vi "Extract subclasses from temperature device.vi"(9 "Data In":string, 10 "Class":string, 11 "Temperature Device Settings in":T1) -> (1 "Data out":string, 3 "Temperature Device Settings out":T1)   [LabVIEW 2014, in "Mercury iXX.lvlib" / "Temperature.lvlib"]
uses:
  Temperature.lvlib
  Controls/Temperature Device (Read).ctl
  Controls/Manufacturing Data.ctl
  Controls/Temperature Sensor Type.ctl
  Controls/Excitation Cluster.ctl
  Controls/Excitation Type.ctl
  Controls/Calibration Cluster.ctl
  Controls/Calibration Interpolation.ctl
  Controls/Loop Cluster.ctl
  Controls/Temperature Signals Cluster.ctl
  Mercury iXX.lvlib
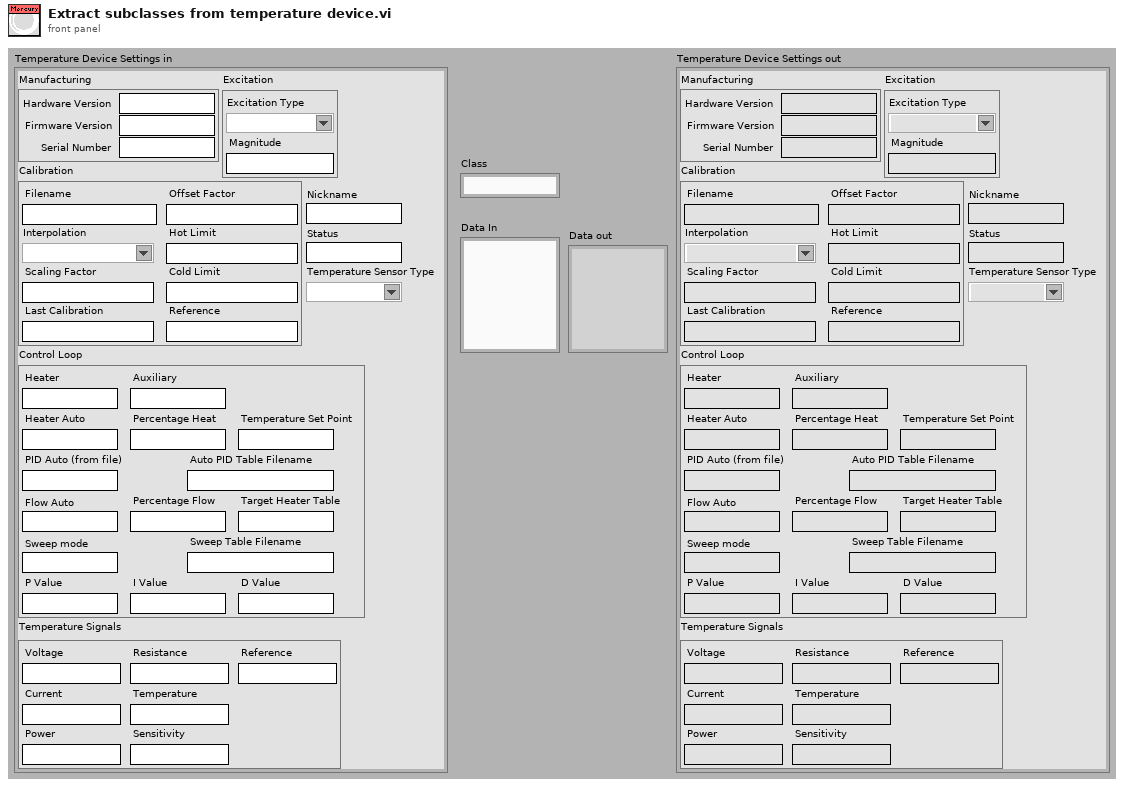
[diagram p1: front panel]
types:
  T1 = typedef "Mercury iXX.lvlib/Temperature.lvlib/Temperature Device (Read).ctl" = cluster{"Manufacturing":T2, "Temperature Sensor Type":T3, "Excitation":T4, "Calibration":T6, "Control Loop":T8, "Temperature Signals":T9, "Nickname":string, "Status":string}
  T2 = typedef "Mercury iXX.lvlib/Manufacturing Data.ctl" = cluster{"Hardware Version":string, "Firmware Version":string, "Serial Number":string}
  T3 = typedef "Mercury iXX.lvlib/Temperature.lvlib/Temperature Sensor Type.ctl" = string
  T4 = typedef "Mercury iXX.lvlib/Temperature.lvlib/Excitation Cluster.ctl" = cluster{"Excitation Type":T5, "Magnitude":string}
  T5 = typedef "Mercury iXX.lvlib/Temperature.lvlib/Excitation Type.ctl" = string
  T6 = typedef "Mercury iXX.lvlib/Temperature.lvlib/Calibration Cluster.ctl" = cluster{"Filename":string, "Interpolation":T7, "Scaling Factor":string, "Offset Factor":string, "Hot Limit":string, "Cold Limit":string, "Last Calibration":string, "Reference":string}
  T7 = typedef "Mercury iXX.lvlib/Temperature.lvlib/Calibration Interpolation.ctl" = string
  T8 = typedef "Mercury iXX.lvlib/Temperature.lvlib/Loop Cluster.ctl" = cluster{"Heater":string, "Auxiliary":string, "Heater Auto":string, "Percentage Heat":string, "Temperature Set Point":string, "PID Auto (from file)":string, "P Value":string, "I Value":string, "D Value":string, "Auto PID Table Filename":string, "Flow Auto":string, "Target Heater Table":string, "Sweep mode":string, "Sweep Table Filename":string, "Percentage Flow":string}
  T9 = typedef "Mercury iXX.lvlib/Temperature.lvlib/Temperature Signals Cluster.ctl" = cluster{"Voltage":string, "Current":string, "Power":string, "Resistance":string, "Temperature":string, "Sensitivity":string, "Reference":string}
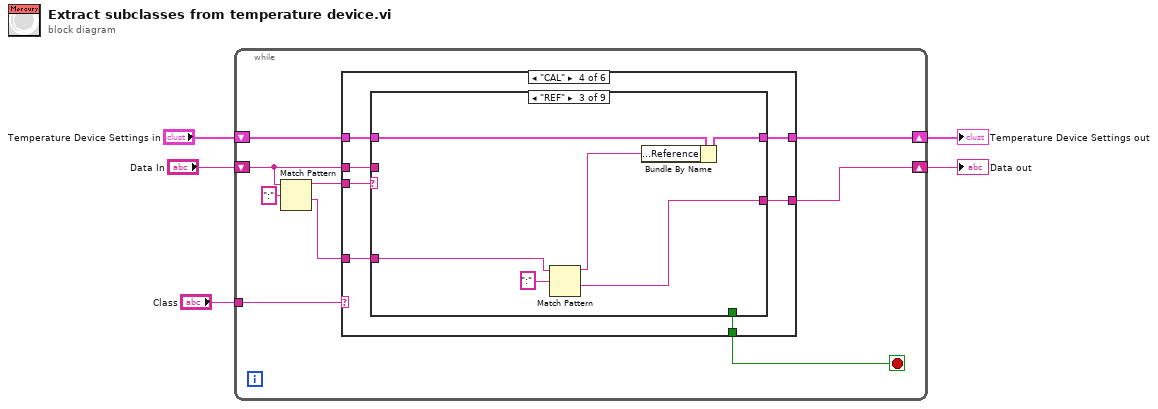
[diagram p0: block diagram]
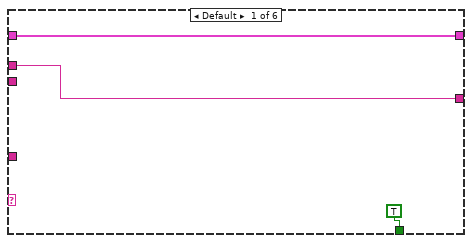
[diagram p2: hidden frame]
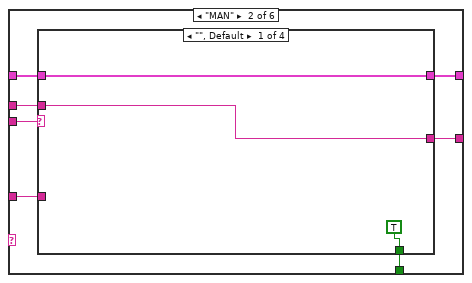
[diagram p3: hidden frame]
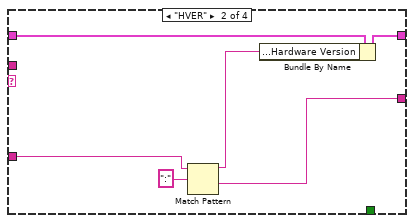
[diagram p4: hidden frame]
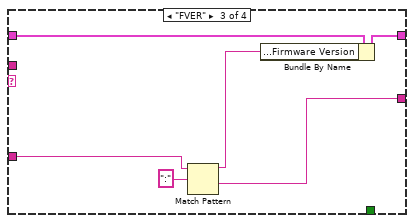
[diagram p5: hidden frame]
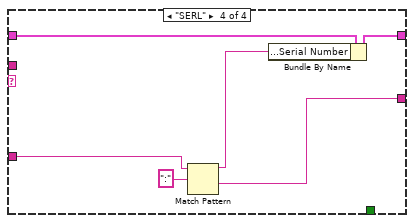
[diagram p6: hidden frame]
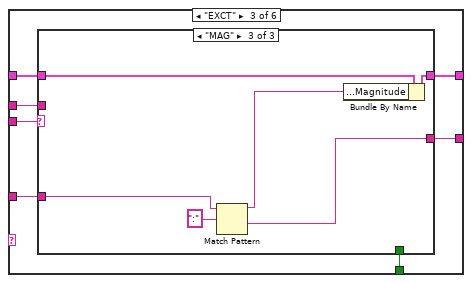
[diagram p7: hidden frame]
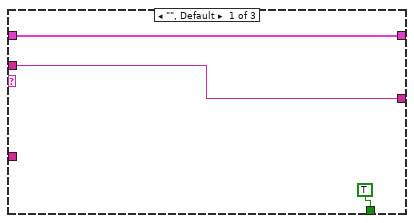
[diagram p8: hidden frame]
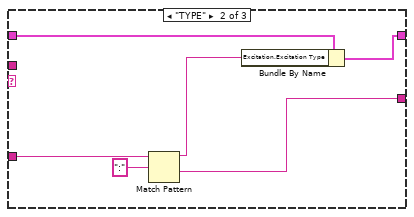
[diagram p9: hidden frame]
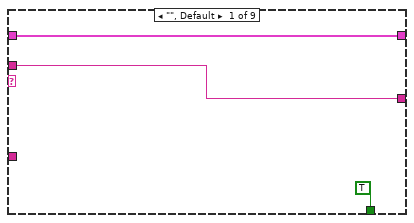
[diagram p10: hidden frame]
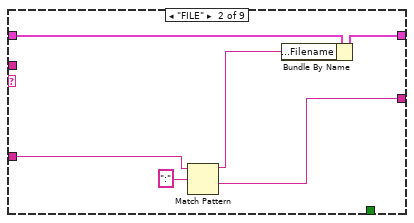
[diagram p11: hidden frame]
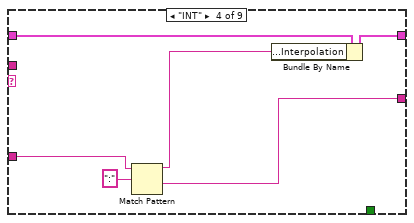
[diagram p12: hidden frame]
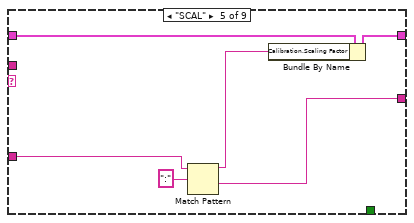
[diagram p13: hidden frame]
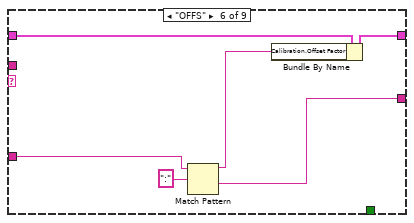
[diagram p14: hidden frame]
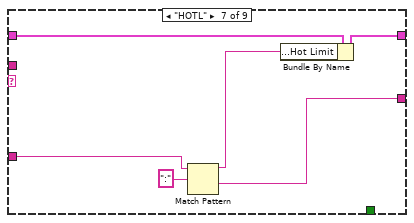
[diagram p15: hidden frame]
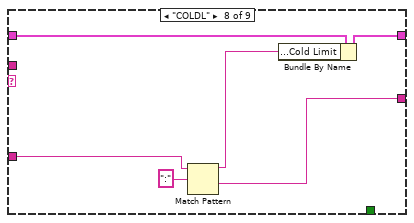
[diagram p16: hidden frame]
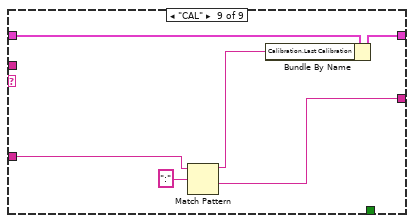
[diagram p17: hidden frame]
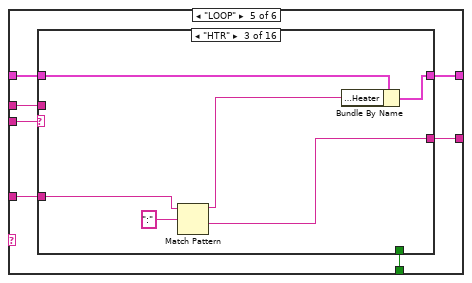
[diagram p18: hidden frame]
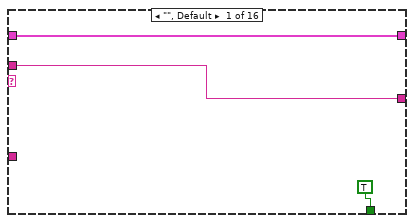
[diagram p19: hidden frame]
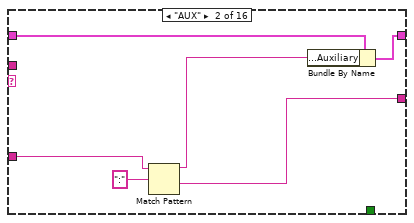
[diagram p20: hidden frame]
diagram:
  n1 = while {
    tunnel: "Class" -> [w7]
    shift-right: [w10] -> w4
    shift-left: "Data In" -> [w8]
    shift-right: [w12] -> w3
    shift-left: "Temperature Device Settings in" -> [w13]
    stop <- w6 stop-if-true
    n2 = Match Pattern(string=w8, regular expression=":") -> (before substring=w9:string, after substring=w11:string)  [unwired: 3 out]
    n3 = case shown="\"CAL\"" w7 {
      tunnel: w13 -> [w17 w24 w52 w74 w132 w232]
      tunnel: [w17 w23 w51 w73 w131 w231] -> w12
      tunnel: w11 -> [_ w22 w50 w72 w130 w230]
      tunnel: [w16 w21 w49 w71 w129 w229] -> w10
      tunnel: w9 -> [_ w20 w48 w70 w128 w228]
      tunnel: w8 -> [w16 w19 w47 w69 w127 w227]
      tunnel: [TRUE w18 w46 w68 w126 w226] -> w6
      frame Default {
      }
      frame "MAN" {
        n4 = case shown="\"\", Default" w20 {
          tunnel: w24 -> [w27 w33 w39 w45]
          tunnel: [w27 w32 w38 w44] -> w23
          tunnel: w22 -> [_ w31 w37 w43]
          tunnel: [w26 w30 w36 w42] -> w21
          tunnel: w19 -> [w26 _ _ _]
          tunnel: [TRUE _ _ _] -> w18
          frame "", Default {
          }
          frame "HVER" {
            n5 = Match Pattern(string=w31, regular expression=":") -> (before substring=w28:string, after substring=w30:string)  [unwired: 3 out]
            n6 = Bundle By Name(cluster=w33, "Manufacturing.Hardware Version"=w28) -> (w32:T1)
          }
          frame "FVER" {
            n7 = Match Pattern(string=w37, regular expression=":") -> (before substring=w34:string, after substring=w36:string)  [unwired: 3 out]
            n8 = Bundle By Name(cluster=w39, "Manufacturing.Firmware Version"=w34) -> (w38:T1)
          }
          frame "SERL" {
            n9 = Match Pattern(string=w43, regular expression=":") -> (before substring=w40:string, after substring=w42:string)  [unwired: 3 out]
            n10 = Bundle By Name(cluster=w45, "Manufacturing.Serial Number"=w40) -> (w44:T1)
          }
        }
      }
      frame "EXCT" {
        n11 = case shown="\"MAG\"" w48 {
          tunnel: w52 -> [w55 w61 w67]
          tunnel: [w55 w60 w66] -> w51
          tunnel: w50 -> [_ w58 w65]
          tunnel: [w54 w57 w64] -> w49
          tunnel: w47 -> [w54 _ _]
          tunnel: [TRUE _ _] -> w46
          frame "", Default {
          }
          frame "TYPE" {
            n12 = Match Pattern(string=w58, regular expression=":") -> (before substring=w56:string, after substring=w57:string)  [unwired: 3 out]
            n13 = Bundle By Name(cluster=w61, "Excitation.Excitation Type"=w56) -> (w60:T1)
          }
          frame "MAG" {
            n14 = Match Pattern(string=w65, regular expression=":") -> (before substring=w62:string, after substring=w64:string)  [unwired: 3 out]
            n15 = Bundle By Name(cluster=w67, "Excitation.Magnitude"=w62) -> (w66:T1)
          }
        }
      }
      frame "CAL" {
        n16 = case shown="\"REF\"" w70 {
          tunnel: w74 -> [w77 w83 w89 w95 w101 w107 w113 w119 w125]
          tunnel: [w77 w82 w88 w94 w100 w106 w112 w118 w124] -> w73
          tunnel: w72 -> [_ w81 w87 w93 w99 w105 w111 w117 w123]
          tunnel: [w76 w80 w86 w92 w98 w104 w110 w116 w122] -> w71
          tunnel: w69 -> [w76 _ _ _ _ _ _ _ _]
          tunnel: [TRUE _ _ _ _ _ _ _ _] -> w68
          frame "", Default {
          }
          frame "FILE" {
            n17 = Match Pattern(string=w81, regular expression=":") -> (before substring=w78:string, after substring=w80:string)  [unwired: 3 out]
            n18 = Bundle By Name(cluster=w83, "Calibration.Filename"=w78) -> (w82:T1)
          }
          frame "REF" {
            n19 = Match Pattern(string=w87, regular expression=":") -> (before substring=w84:string, after substring=w86:string)  [unwired: 3 out]
            n20 = Bundle By Name(cluster=w89, "Calibration.Reference"=w84) -> (w88:T1)
          }
          frame "INT" {
            n21 = Match Pattern(string=w93, regular expression=":") -> (before substring=w90:string, after substring=w92:string)  [unwired: 3 out]
            n22 = Bundle By Name(cluster=w95, "Calibration.Interpolation"=w90) -> (w94:T1)
          }
          frame "SCAL" {
            n23 = Match Pattern(string=w99, regular expression=":") -> (before substring=w96:string, after substring=w98:string)  [unwired: 3 out]
            n24 = Bundle By Name(cluster=w101, "Calibration.Scaling Factor"=w96) -> (w100:T1)
          }
          frame "OFFS" {
            n25 = Match Pattern(string=w105, regular expression=":") -> (before substring=w102:string, after substring=w104:string)  [unwired: 3 out]
            n26 = Bundle By Name(cluster=w107, "Calibration.Offset Factor"=w102) -> (w106:T1)
          }
          frame "HOTL" {
            n27 = Match Pattern(string=w111, regular expression=":") -> (before substring=w108:string, after substring=w110:string)  [unwired: 3 out]
            n28 = Bundle By Name(cluster=w113, "Calibration.Hot Limit"=w108) -> (w112:T1)
          }
          frame "COLDL" {
            n29 = Match Pattern(string=w117, regular expression=":") -> (before substring=w114:string, after substring=w116:string)  [unwired: 3 out]
            n30 = Bundle By Name(cluster=w119, "Calibration.Cold Limit"=w114) -> (w118:T1)
          }
          frame "CAL" {
            n31 = Match Pattern(string=w123, regular expression=":") -> (before substring=w120:string, after substring=w122:string)  [unwired: 3 out]
            n32 = Bundle By Name(cluster=w125, "Calibration.Last Calibration"=w120) -> (w124:T1)
          }
        }
      }
      frame "LOOP" {
        n33 = case shown="\"HTR\"" w128 {
          tunnel: w132 -> [w135 w141 w147 w153 w159 w165 w171 w177 w183 w189 w195 w201 w207 w213 w219 w225]
          tunnel: [w135 w140 w146 w152 w158 w164 w170 w176 w182 w188 w194 w200 w206 w212 w218 w224] -> w131
          tunnel: w130 -> [_ w138 w144 w150 w156 w162 w168 w174 w181 w187 w193 w199 w205 w211 w217 w223]
          tunnel: [w134 w137 w143 w149 w155 w161 w167 w173 w180 w186 w192 w198 w204 w210 w216 w222] -> w129
          tunnel: w127 -> [w134 _ _ _ _ _ _ _ _ _ _ _ _ _ _ _]
          tunnel: [TRUE _ _ _ _ _ _ _ _ _ _ _ _ _ _ _] -> w126
          frame "", Default {
          }
          frame "AUX" {
            n34 = Match Pattern(string=w138, regular expression=":") -> (before substring=w136:string, after substring=w137:string)  [unwired: 3 out]
            n35 = Bundle By Name(cluster=w141, "Control Loop.Auxiliary"=w136) -> (w140:T1)
          }
          frame "HTR" {
            n36 = Match Pattern(string=w144, regular expression=":") -> (before substring=w142:string, after substring=w143:string)  [unwired: 3 out]
            n37 = Bundle By Name(cluster=w147, "Control Loop.Heater"=w142) -> (w146:T1)
          }
          frame "ENAB" {
            n38 = Match Pattern(string=w150, regular expression=":") -> (before substring=w148:string, after substring=w149:string)  [unwired: 3 out]
            n39 = Bundle By Name(cluster=w153, "Control Loop.Heater Auto"=w148) -> (w152:T1)
          }
          frame "HSET" {
            n40 = Match Pattern(string=w156, regular expression=":") -> (before substring=w154:string, after substring=w155:string)  [unwired: 3 out]
            n41 = Bundle By Name(cluster=w159, "Control Loop.Percentage Heat"=w154) -> (w158:T1)
          }
          frame "TSET" {
            n42 = Match Pattern(string=w162, regular expression=":") -> (before substring=w160:string, after substring=w161:string)  [unwired: 3 out]
            n43 = Bundle By Name(cluster=w165, "Control Loop.Temperature Set Point"=w160) -> (w164:T1)
          }
          frame "PIDT" {
            n44 = Match Pattern(string=w168, regular expression=":") -> (before substring=w166:string, after substring=w167:string)  [unwired: 3 out]
            n45 = Bundle By Name(cluster=w171, "Control Loop.PID Auto (from file)"=w166) -> (w170:T1)
          }
          frame "PIDF" {
            n46 = Match Pattern(string=w174, regular expression=":") -> (before substring=w172:string, after substring=w173:string)  [unwired: 3 out]
            n47 = Bundle By Name(cluster=w177, "Control Loop.Auto PID Table Filename"=w172) -> (w176:T1)
          }
          frame "P" {
            n48 = Match Pattern(string=w181, regular expression=":") -> (before substring=w178:string, after substring=w180:string)  [unwired: 3 out]
            n49 = Bundle By Name(cluster=w183, "Control Loop.P Value"=w178) -> (w182:T1)
          }
          frame "I" {
            n50 = Match Pattern(string=w187, regular expression=":") -> (before substring=w184:string, after substring=w186:string)  [unwired: 3 out]
            n51 = Bundle By Name(cluster=w189, "Control Loop.I Value"=w184) -> (w188:T1)
          }
          frame "D" {
            n52 = Match Pattern(string=w193, regular expression=":") -> (before substring=w190:string, after substring=w192:string)  [unwired: 3 out]
            n53 = Bundle By Name(cluster=w195, "Control Loop.D Value"=w190) -> (w194:T1)
          }
          frame "FAUT" {
            n54 = Match Pattern(string=w199, regular expression=":") -> (before substring=w196:string, after substring=w198:string)  [unwired: 3 out]
            n55 = Bundle By Name(cluster=w201, "Control Loop.Flow Auto"=w196) -> (w200:T1)
          }
          frame "FSET" {
            n56 = Match Pattern(string=w205, regular expression=":") -> (before substring=w202:string, after substring=w204:string)  [unwired: 3 out]
            n57 = Bundle By Name(cluster=w207, "Control Loop.Percentage Flow"=w202) -> (w206:T1)
          }
          frame "THTF" {
            n58 = Match Pattern(string=w211, regular expression=":") -> (before substring=w208:string, after substring=w210:string)  [unwired: 3 out]
            n59 = Bundle By Name(cluster=w213, "Control Loop.Target Heater Table"=w208) -> (w212:T1)
          }
          frame "SWMD" {
            n60 = Match Pattern(string=w217, regular expression=":") -> (before substring=w214:string, after substring=w216:string)  [unwired: 3 out]
            n61 = Bundle By Name(cluster=w219, "Control Loop.Sweep mode"=w214) -> (w218:T1)
          }
          frame "SWFL" {
            n62 = Match Pattern(string=w223, regular expression=":") -> (before substring=w220:string, after substring=w222:string)  [unwired: 3 out]
            n63 = Bundle By Name(cluster=w225, "Control Loop.Sweep Table Filename"=w220) -> (w224:T1)
          }
        }
      }
      frame "SIG" {
        n64 = case shown="\"TEMP\"" w228 {
          tunnel: w232 -> [w235 w241 w247 w253 w259 w265 w271 w277]
          tunnel: [w235 w240 w246 w252 w258 w264 w270 w276] -> w231
          tunnel: w230 -> [_ w239 w245 w251 w257 w263 w269 w275]
          tunnel: [w234 w238 w244 w250 w256 w262 w268 w274] -> w229
          tunnel: w227 -> [w234 _ _ _ _ _ _ _]
          tunnel: [TRUE _ _ _ _ _ _ _] -> w226
          frame "", Default {
          }
          frame "VOLT" {
            n65 = Match Pattern(string=w239, regular expression=":") -> (before substring=w236:string, after substring=w238:string)  [unwired: 3 out]
            n66 = Bundle By Name(cluster=w241, "Temperature Signals.Voltage"=w236) -> (w240:T1)
          }
          frame "CURR" {
            n67 = Match Pattern(string=w245, regular expression=":") -> (before substring=w242:string, after substring=w244:string)  [unwired: 3 out]
            n68 = Bundle By Name(cluster=w247, "Temperature Signals.Current"=w242) -> (w246:T1)
          }
          frame "POWR" {
            n69 = Match Pattern(string=w251, regular expression=":") -> (before substring=w248:string, after substring=w250:string)  [unwired: 3 out]
            n70 = Bundle By Name(cluster=w253, "Temperature Signals.Power"=w248) -> (w252:T1)
          }
          frame "RES" {
            n71 = Match Pattern(string=w257, regular expression=":") -> (before substring=w254:string, after substring=w256:string)  [unwired: 3 out]
            n72 = Bundle By Name(cluster=w259, "Temperature Signals.Resistance"=w254) -> (w258:T1)
          }
          frame "TEMP" {
            n73 = Match Pattern(string=w263, regular expression=":") -> (before substring=w260:string, after substring=w262:string)  [unwired: 3 out]
            n74 = Bundle By Name(cluster=w265, "Temperature Signals.Temperature"=w260) -> (w264:T1)
          }
          frame "SLOP" {
            n75 = Match Pattern(string=w269, regular expression=":") -> (before substring=w266:string, after substring=w268:string)  [unwired: 3 out]
            n76 = Bundle By Name(cluster=w271, "Temperature Signals.Sensitivity"=w266) -> (w270:T1)
          }
          frame "REF" {
            n77 = Match Pattern(string=w275, regular expression=":") -> (before substring=w272:string, after substring=w274:string)  [unwired: 3 out]
            n78 = Bundle By Name(cluster=w277, "Temperature Signals.Reference"=w272) -> (w276:T1)
          }
        }
      }
    }
  }
  "Data out" <- w4
  "Temperature Device Settings out" <- w3
